vi "subLoadBlacklist.vi"() -> (0 "error out":errorcluster, 2 "Blacklist":T1[](array[typedef]))   [LabVIEW 2014, in "lvbuildsecurity.lvlib"]
uses:
  lvbuildsecurity.lvlib
  ctlBlacklistClass.ctl
  <vilib>/Utility/config.llb/Read Key (String).vi
  <vilib>/Utility/config.llb/NI_LVConfig.lvlib
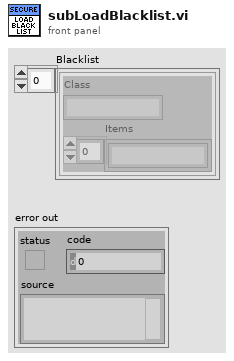
[diagram p1: front panel]
types:
  T1 = typedef "lvbuildsecurity.lvlib/ctlBlacklistClass.ctl" = cluster{"Class":string, "Items":string[]}
  T2 = typedef "NI_LVConfig.lvlib/Config Data RefNum.ctl" = refnum<k1>
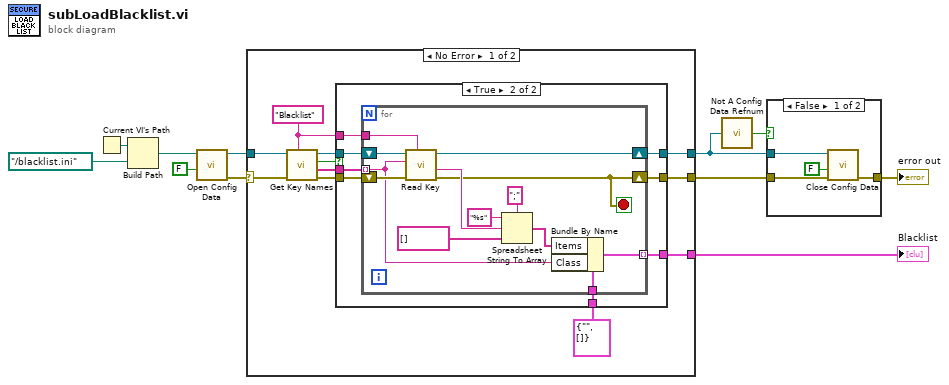
[diagram p0: block diagram]
diagram:
  n1 = Current VI's Path() -> (path=w10:path)
  n2 = Build Path(base path=w10, name or relative path=path "../blacklist.ini" ("configuration file path")) -> (appended path=w8:path)
  n3 = call <vilib>:"Open Config Data.vi"("create file if necessary (T)"=FALSE, "configuration file path"=w8) -> ("error out"=w5:errorcluster, "refnum"=w7:T2)  [unwired: 7 in, 1 out]
  n4 = case shown="No Error" w5 {
    selector: w5 -> [w14 _]
    tunnel: w7 -> [w22 w46]
    tunnel: [w15 _] -> w6
    tunnel: [w13 _] -> w4
    tunnel: [w12 w46] -> w3
    frame No Error {
      w17 = "Blacklist" ("section")
      n5 = call <vilib>:"Get Key Names.vi"("section"=w17, "error in (no error)"=w14, "refnum"=w22) -> ("error out"=w21:errorcluster, "key names"=w19:string[], "section exists?"=w18:bool, "refnum out"=w20:T2)  [unwired: 5 in]
      n6 = case shown="True" w18 {
        tunnel: w21 -> [w23 w32]
        tunnel: w20 -> [w24 w31]
        tunnel: w19 -> [_ w30]
        tunnel: w17 -> [_ w29]
        tunnel: T1 {"Class"="", "Items"=[]} ("Blacklist Class") -> [_ w28]
        tunnel: [_ w27] -> w15
        tunnel: [w23 w26] -> w13
        tunnel: [w24 w25] -> w12
        frame False {
        }
        frame True {
          n7 = for {
            shift-right: [w33] -> w26
            shift-left: w32 -> [w45]
            shift-right: [w42] -> w25
            shift-left: w31 -> [w44]
            tunnel: w30 -> [w34] mode=indexing
            tunnel: w29 -> [w43]
            tunnel: w28 -> [w41]
            tunnel: [w36] -> w27 mode=indexing
            stop <- w33 stop-if-true
            n8 = call-poly <vilib>:"Read Key.vi"("section"=w43, "error in (no error)"=w45, "key"=w34, "refnum"=w44) -> ("error out"=w33:errorcluster, "value"=w40:string, "refnum out"=w42:T2)  [unwired: 4 in, 1 out]
            n9 = Spreadsheet String To Array(delimiter (Tab)=";", format string="%s", spreadsheet string=w40, array type (2D Dbl)=string[] []) -> (array=w35:string[])
            n10 = Bundle By Name(cluster=w41, "Items"=w35, "Class"=w34) -> (w36:T1)
          }
        }
      }
    }
    frame Error {
      # "Allow anything if blacklist doesn't exist."
    }
  }
  "Blacklist" <- w6
  n11 = call <vilib>:"Not A Config Data Refnum.vi"("refnum"=w3) -> ("not a config data refnum"=w2:bool)
  n12 = case shown="False" w2 {
    tunnel: w3 -> [w50 _]
    tunnel: w4 -> [w49 w51]
    tunnel: [w48 w51] -> w1
    frame False {
      n13 = call <vilib>:"Close Config Data.vi"("error in (no error)"=w49, "write file if changed (T)"=FALSE ("create file if necessary (T)"), "refnum"=w50) -> ("error out"=w48:errorcluster)  [unwired: 7 in, 1 out]
    }
    frame True {
    }
  }
  "error out" <- w1
